vi "Set Type.vi"(10 "Type":refnum<class "Type.lvclass">, 11 "BooleanPanel in":refnum<class "BooleanPanel.lvclass">) -> (3 "BooleanPanel out":refnum<class "BooleanPanel.lvclass">)   [LabVIEW 2020, in "Conditum-Tools.lvlib" / "BooleanPanel.lvclass"]
uses:
  BooleanPanel.lvclass
  Conditum-Clone/Columns/Type/Type.lvclass
  BooleanPanel.lvclass/BooleanPanel.ctl
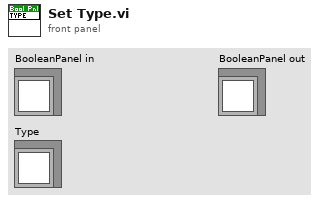
[diagram p1: front panel]
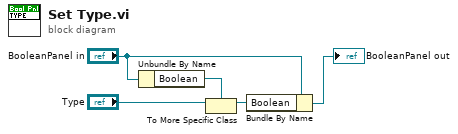
[diagram p0: block diagram]
diagram:
  n1 = Unbundle By Name("BooleanPanel in") -> ("Boolean"=w1:refnum<class "Boolean.lvclass">)
  n2 = To More Specific Class(target class=w1, reference="Type") -> (specific class reference=w4:refnum<class "Boolean.lvclass">)  [unwired: 1 in, 1 out]
  n3 = Bundle By Name(cluster="BooleanPanel in", "Boolean"=w4) -> (→"BooleanPanel out":refnum<class "BooleanPanel.lvclass">)
